vi "Translate.vi"(0 "reference":refnum<class "ClassRelationshipEdge.lvclass">, 1 "dx":dbl format="%.2f", 2 "dy":dbl format="%.2f", 3 "StartEndNode":refnum<class "AbstractNode.lvclass">, 5 "error in (no error)":errorcluster) -> (14 "reference out":refnum<class "ClassRelationshipEdge.lvclass">, 19 "error out":errorcluster)   [LabVIEW 2016, in "ClassRelationshipEdge.lvclass"]
uses:
  <resource>/Framework/Providers/Open_GDS/UML/ClassRelationshipEdge_class/ClassRelationshipEdge.lvclass
  C:/Program Files (x86)/National Instruments/LabVIEW 2016/resource/Framework/Providers/Open_GDS/UML/SegmentedLineEdge_class/SegmentedLineEdge.lvclass
  C:/Program Files (x86)/National Instruments/LabVIEW 2016/resource/Framework/Providers/Open_GDS/UML/AbstractEdge_class/AbstractEdge.lvclass
  <resource>/Framework/Providers/Open_GDS/UML/AbstractNode_class/AbstractNode.lvclass
  <resource>/Framework/Providers/Open_GDS/UML/SegmentedLineEdge_class/SegmentedLineEdge.lvclass
  <resource>/Framework/Providers/Open_GDS/UML/AbstractEdge_class/AbstractEdge.lvclass
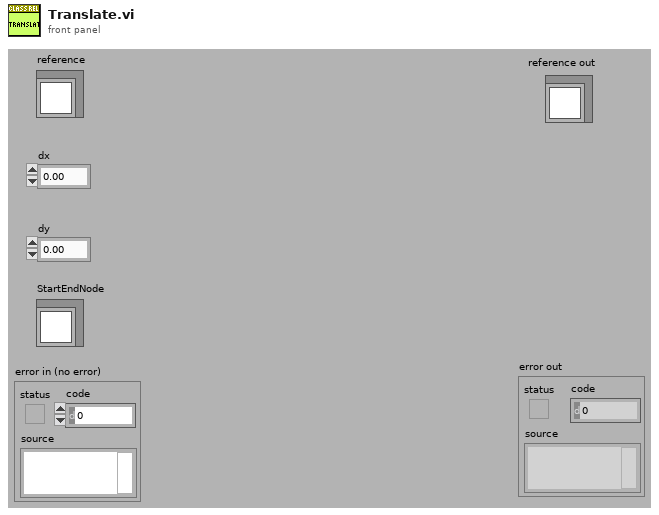
[diagram p1: front panel]
types:
  T1 = typedef "Rectangle Rectangle2D.ctl" = cluster{"x":dbl, "y":dbl, "width":dbl, "height":dbl}
  T2 = typedef "AbstractEdge.lvclass/ObjectAttributes.ctl" = cluster{"start":refnum<class "AbstractNode.lvclass">, "end":refnum<class "AbstractNode.lvclass">}
  T3 = typedef "ClassRelationshipEdge.lvclass/ObjectAttributes.ctl" = cluster{"bentStyleRef":refnum<class "BentStyle.lvclass">, "startConnectionOffset":cluster{"x":i32, "y":i32}, "endConnectionOffset":cluster{"x":i32, "y":i32}, "MidLineOffset":cluster{"x":i32, "y":i32}, "DepClass":T4}
  T4 = typedef "ReversedEngineering_ViDependencyDetailsType.ctl" = cluster{"ThisVIs/Ctls":path[], "Dependent_VIs/Ctls":path[]}
  T5 = typedef "Point Point2D.ctl" = cluster{"x":dbl, "y":dbl}
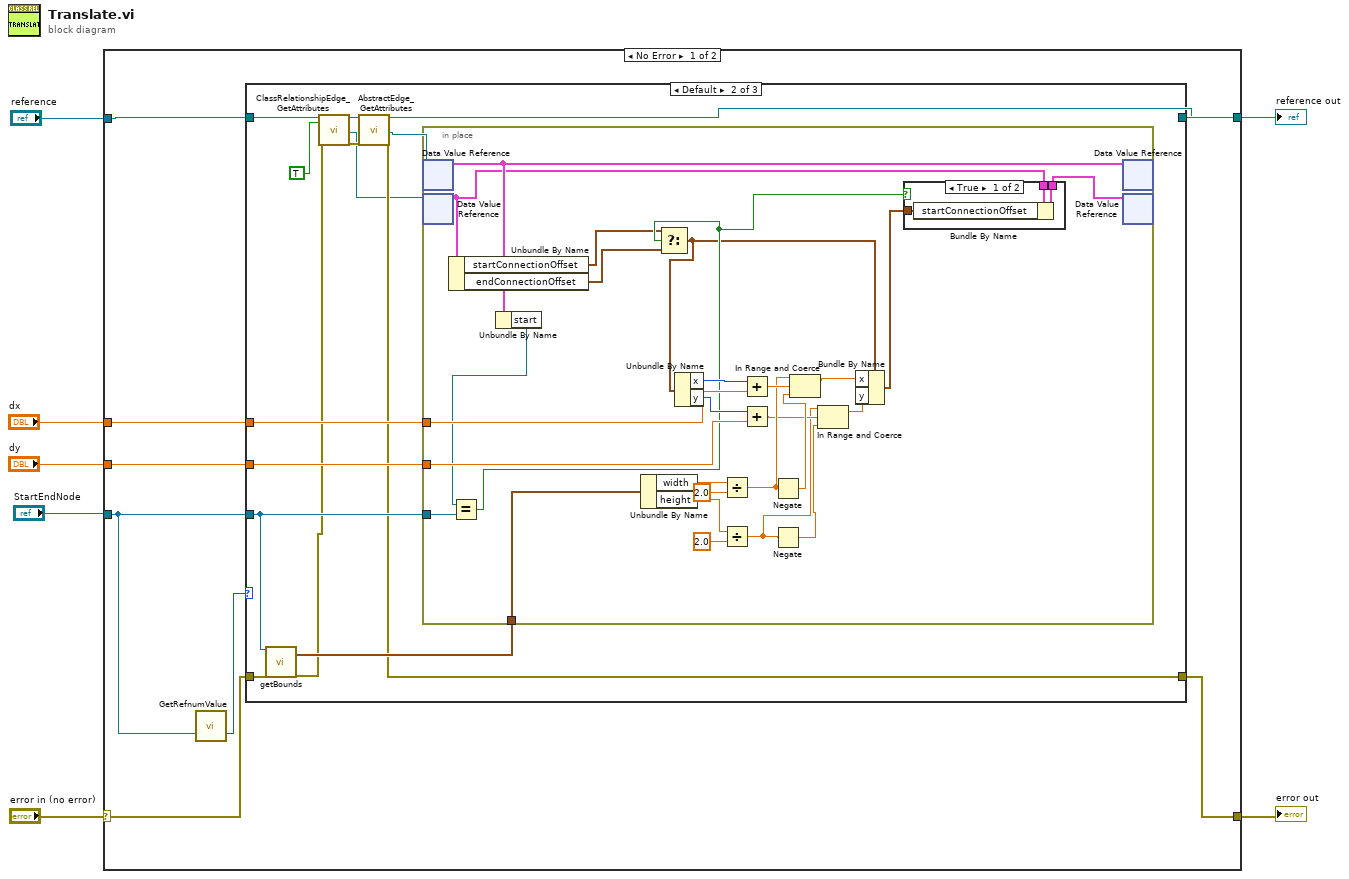
[diagram p0: block diagram]
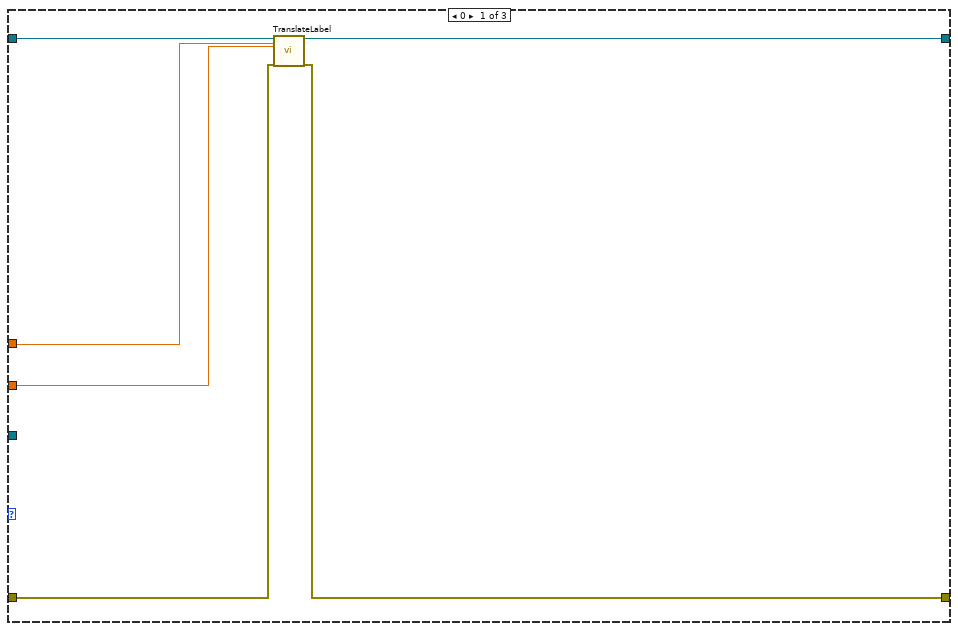
[diagram p2: hidden frame]
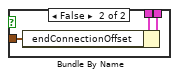
[diagram p3: hidden frame]
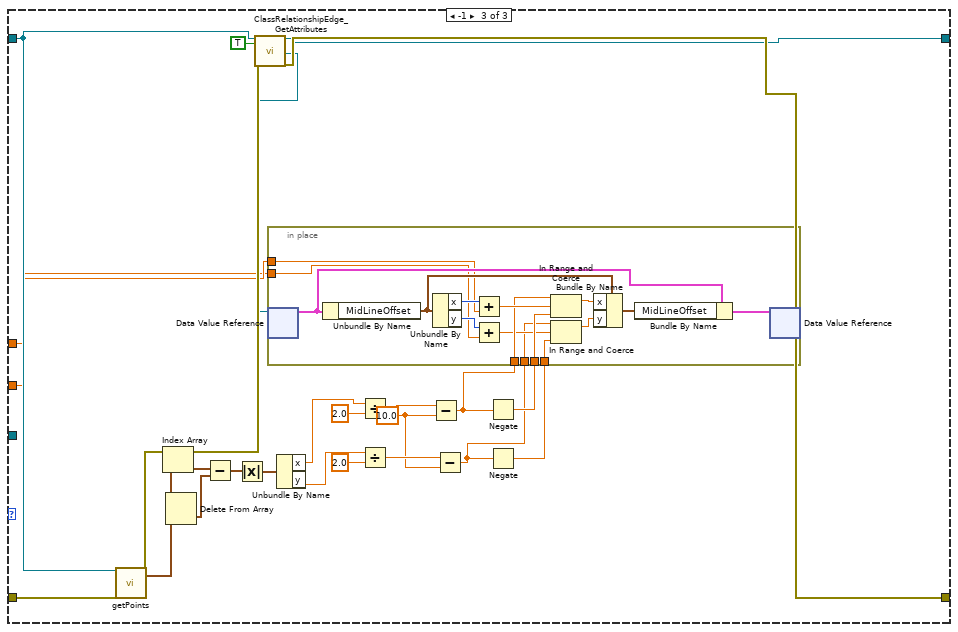
[diagram p4: hidden frame]
diagram:
  n1 = case shown="No Error" "error in (no error)" {
    selector: "error in (no error)" -> [w15 w110]
    tunnel: "reference" -> [w14 w111]
    tunnel: [w13 w110] -> w5
    tunnel: [w12 w111] -> w4
    tunnel: "StartEndNode" -> [w9 _]
    tunnel: "dx" -> [w11 _]
    tunnel: "dy" -> [w10 _]
    frame No Error {
      n2 = call <resource>:"GetRefnumValue.vi"("reference"=w9) -> ("RefNum"=w8:i32)  [unwired: 17 in, 1 out]
      n3 = case shown="Default" w8 {
        tunnel: w15 -> [w18 w26 w88]
        tunnel: w14 -> [w21 w35 w86]
        tunnel: [w17 w24 w93] -> w13
        tunnel: [w16 w34 w92] -> w12
        tunnel: w11 -> [w20 w33 w70]
        tunnel: w10 -> [w19 w32 w69]
        tunnel: w9 -> [_ w30 _]
        frame 0 {
          n4 = call <resource>:"TranslateLabel.vi"("reference"=w21, "dx"=w20, "dy"=w19, "error in (no error)"=w18) -> ("reference out"=w16:refnum<class "ClassRelationshipEdge.lvclass">, "error out"=w17:errorcluster)  [unwired: 1 in, 13 out]
        }
        frame Default {
          n5 = call-dynamic "getBounds.vi"("reference"=w30, "error in (no error)"=w26) -> ("bounds"=w31:T1, "error out"=w25:errorcluster)  [unwired: 15 in, 1 out]
          n6 = call <resource>:"ClassRelationshipEdge_GetAttributes.vi"("reference in"=w35, "OnlyGetDvrReference(False)"=TRUE, "error in (no error)"=w25) -> ("reference out"=w28:refnum<class "ClassRelationshipEdge.lvclass">, "DataRef"=w22:refnum<data-value>, "error out"=w27:errorcluster)  [unwired: 13 in, 1 out]
          n7 = call <resource>:"AbstractEdge_GetAttributes.vi"("reference in"=w28, "error in (no error)"=w27) -> ("reference out"=w34:refnum<class "ClassRelationshipEdge.lvclass">, "DataRef"=w23:refnum<data-value>, "error out"=w24:errorcluster)  [unwired: 14 in, 1 out]
          n8 = in-place {
            in-place-border: w33 -> [w62]
            in-place-border: w32 -> [w60]
            in-place-border: w31 -> [w59]
            in-place-border: w30 -> [w42]
            n9 = in-place-dvr #1(w23) -> (w38:T2)  [unwired: 1 out]
            n10 = in-place-dvr #2(w22) -> (w37:T3)  [unwired: 1 out]
            n11 = Unbundle By Name(w37) -> ("startConnectionOffset"=w41:cluster{"x":i32, "y":i32}, "endConnectionOffset"=w40:cluster{"x":i32, "y":i32})
            n12 = Unbundle By Name(w38) -> ("start"=w39:refnum<class "AbstractNode.lvclass">)
            n13 = Equal?(x=w39, y=w42) -> (x = y?=w47:bool)
            n14 = Unbundle By Name(w59) -> ("width"=w57:dbl, "height"=w51:dbl)
            n15 = Select(t=w41, s=w47, f=w40) -> (s? t:f=w46:cluster{"x":i32, "y":i32})
            n16 = Unbundle By Name(w46) -> ("x"=w48:i32, "y"=w61:i32)
            n17 = Divide(x=w57, y=2.0) -> (x/y=w54:dbl)
            n18 = Divide(x=w51, y=2.0) -> (x/y=w49:dbl)
            n19 = Add(x=w48, y=w62) -> (x+y=w58:dbl)
            n20 = Add(x=w61, y=w60) -> (x+y=w53:dbl)
            n21 = Negate(x=w54) -> (-x=w55:dbl)
            n22 = Negate(x=w49) -> (-x=w50:dbl)
            n23 = In Range and Coerce(upper limit=w54, x=w58, lower limit=w55) -> (coerced(x)=w45:dbl)  [unwired: 1 out]
            n24 = In Range and Coerce(upper limit=w49, x=w53, lower limit=w50) -> (coerced(x)=w44:dbl)  [unwired: 1 out]
            n25 = Bundle By Name(cluster=w46, "x"=w45, "y"=w44) -> (w43:cluster{"x":i32, "y":i32})
            n26 = case shown="True" w47 {
              tunnel: [w65 w68] -> w36
              tunnel: w43 -> [w64 w67]
              tunnel: w37 -> [w63 w66]
              frame True {
                n27 = Bundle By Name(cluster=w63, "startConnectionOffset"=w64) -> (w65:T3)
              }
              frame False {
                n28 = Bundle By Name(cluster=w66, "endConnectionOffset"=w67) -> (w68:T3)
              }
            }
            n29 = in-place-dvr #1(w38) -> ()  [unwired: 2 out]
            n30 = in-place-dvr #2(w36) -> ()  [unwired: 2 out]
          }
        }
        frame -1 {
          w77 = 10.0 ("y")
          n31 = call-dynamic "getPoints.vi"("reference"=w86, "error in (no error)"=w88) -> ("points"=w85:T5[], "error out"=w87:errorcluster)  [unwired: 15 in, 1 out]
          n32 = Index Array(array=w85) -> (element=w84:T5)  [unwired: 1 in]
          n33 = Delete From Array(array=w85) -> (deleted portion=w83:T5)  [unwired: 2 in, 1 out]
          n34 = Subtract(x=w84, y=w83) -> (x-y=w82:T5)
          n35 = Absolute Value(x=w82) -> (abs(x)=w81:T5)
          n36 = call <resource>:"ClassRelationshipEdge_GetAttributes.vi"("reference in"=w86, "OnlyGetDvrReference(False)"=TRUE, "error in (no error)"=w87) -> ("reference out"=w92:refnum<class "ClassRelationshipEdge.lvclass">, "DataRef"=w75:refnum<data-value>, "error out"=w93:errorcluster)  [unwired: 13 in, 1 out]
          n37 = Unbundle By Name(w81) -> ("x"=w80:dbl, "y"=w79:dbl)
          n38 = Divide(x=w80, y=2.0) -> (x/y=w90:dbl)
          n39 = Divide(x=w79, y=2.0) -> (x/y=w78:dbl)
          n40 = Subtract(x=w90, y=w77) -> (x-y=w73:dbl)
          n41 = Subtract(x=w78, y=w77) -> (x-y=w71:dbl)
          n42 = Negate(x=w73) -> (-x=w74:dbl)
          n43 = Negate(x=w71) -> (-x=w72:dbl)
          n44 = in-place {
            in-place-border: w74 -> [w101]
            in-place-border: w73 -> [w99]
            in-place-border: w72 -> [w98]
            in-place-border: w71 -> [w96]
            in-place-border: w70 -> [w95]
            in-place-border: w69 -> [w94]
            n45 = in-place-dvr #3(w75) -> (w109:T3)  [unwired: 1 out]
            n46 = Unbundle By Name(w109) -> ("MidLineOffset"=w106:cluster{"x":i32, "y":i32})
            n47 = Unbundle By Name(w106) -> ("x"=w103:i32, "y"=w102:i32)
            n48 = Add(x=w103, y=w95) -> (x+y=w100:dbl)
            n49 = Add(x=w102, y=w94) -> (x+y=w97:dbl)
            n50 = In Range and Coerce(upper limit=w99, x=w100, lower limit=w101) -> (coerced(x)=w105:dbl)  [unwired: 1 out]
            n51 = In Range and Coerce(upper limit=w96, x=w97, lower limit=w98) -> (coerced(x)=w104:dbl)  [unwired: 1 out]
            n52 = Bundle By Name(cluster=w106, "x"=w105, "y"=w104) -> (w108:cluster{"x":i32, "y":i32})
            n53 = Bundle By Name(cluster=w109, "MidLineOffset"=w108) -> (w107:T3)
            n54 = in-place-dvr #3(w107) -> ()  [unwired: 2 out]
          }
        }
      }
    }
    frame Error {
    }
  }
  "reference out" <- w4
  "error out" <- w5
